vi "WS1050_AD7747_Control_Cap_bank_Measure S0.vi"(0 "Select Com Port":refnum<visa-resource-name>="COM1", 1 "Click down to quit":bool, 2 "Push Button to Initialize AD7747":bool, 3 "Push Button to Calibrate":bool, 7 "Push Button to write Offset":bool, 11 "errorin":errorcluster, 12 "Push Button to Measue Cap":bool=TRUE, 13 "CApDac_values":string[](array[string])=["900b89", "900b89", "900b89"]) -> (4 "C2L(pF)":dbl, 8 "C1L(pF)":dbl, 10 "C3L(pF)":dbl, 14 "Com Port Out":refnum<visa-resource-name>="COM1", 15 "error out":errorcluster)   [LabVIEW 2009]
panel:
  # "AD7747 Control Ver1.0"
  # "Interface PIC I2C Control"
  # "Bank Cap Measurements"
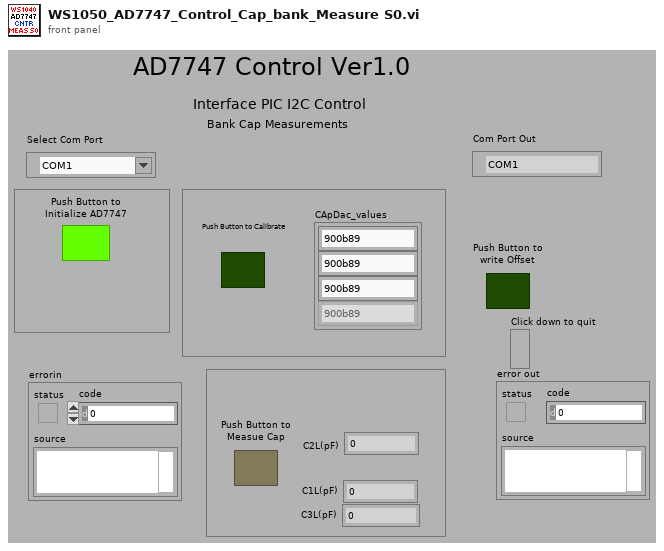
[diagram p1: front panel]
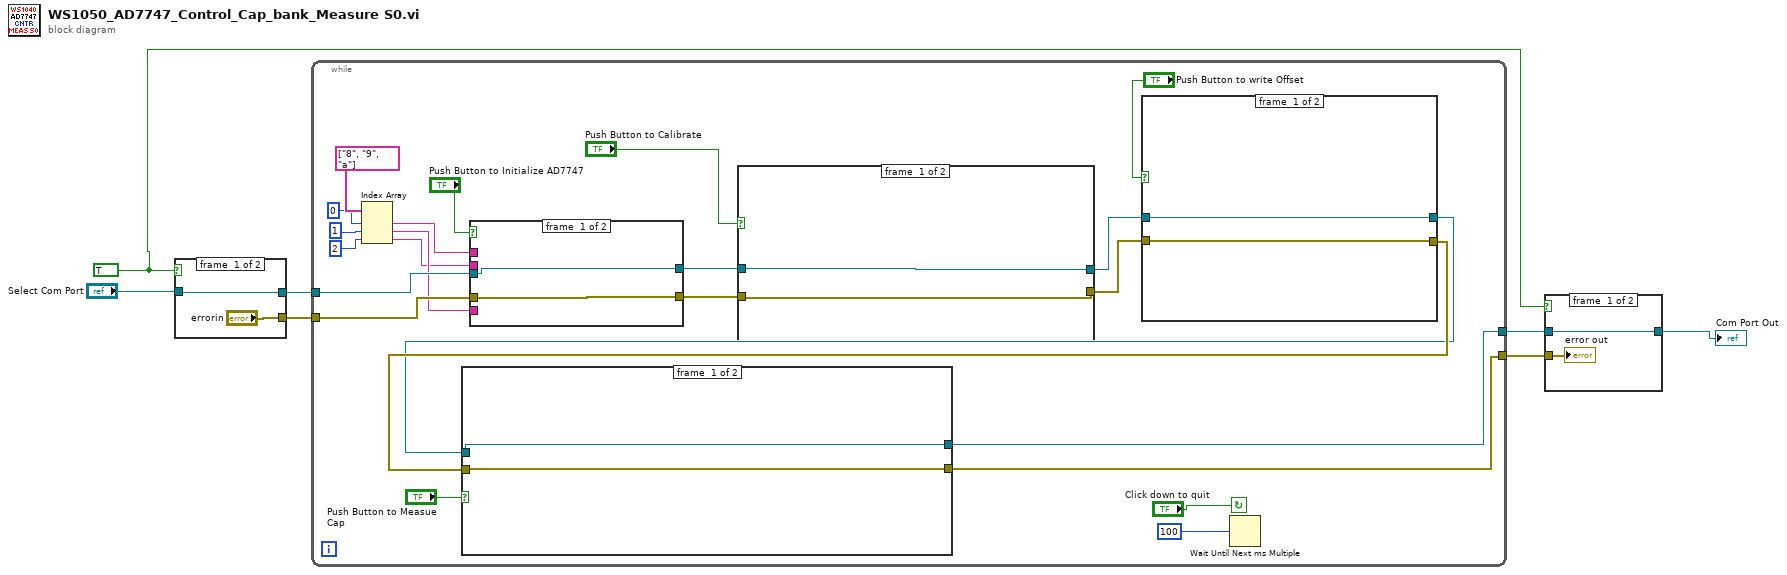
[diagram p0: block diagram]
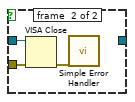
[diagram p2: hidden frame]
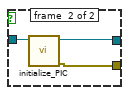
[diagram p3: hidden frame]
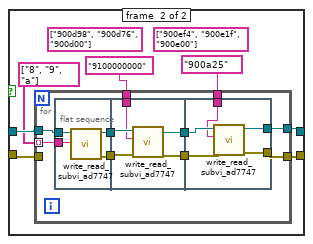
[diagram p4: hidden frame]
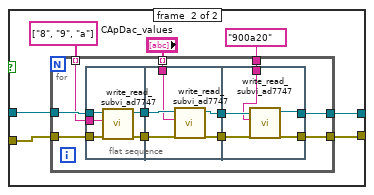
[diagram p5: hidden frame]
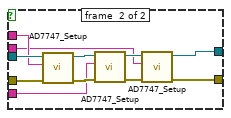
[diagram p6: hidden frame]
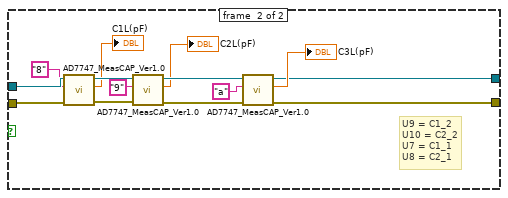
[diagram p7: hidden frame]
diagram:
  w2 = TRUE
  n1 = case shown="True" w2 {
    tunnel: ["errorin" w12] -> w7
    tunnel: [w8 w11] -> w6
    tunnel: "Select Com Port" -> [w8 w10]
    frame #0 {
    }
    frame #1 {
      n2 = call "initialize_PIC.vi"("Select Com Port"=w10) -> ("error out"=w12:errorcluster, "VISA resource name out"=w11:refnum<visa-resource-name>)  [unwired: 9 in]
    }
  }
  n3 = while {
    tunnel: w7 -> [w30]
    tunnel: w6 -> [w28]
    tunnel: [w17] -> w5
    tunnel: [w35] -> w4
    stop <- "Click down to quit" continue-if-true
    n4 = Index Array(array=string[] ["8", "9", "a"], index #1=0 ("index"), index #2=1 ("index"), index #3=2 ("index")) -> (element #1=w31:string, element #2=w24:string, element #3=w23:string)
    n5 = case shown="True" "Push Button to Initialize AD7747" {
      tunnel: w30 -> [w104 w115]
      tunnel: [w104 w105] -> w18
      tunnel: w28 -> [w103 w114]
      tunnel: w31 -> [_ w109]
      tunnel: w24 -> [_ w108]
      tunnel: w23 -> [_ w107]
      tunnel: [w103 w106] -> w15
      frame #0 {
      }
      frame #1 {
        n6 = call "AD7747_Setup.vi"("error in"=w115, "AD7747_Number"=w109, "Control"=w114) -> ("error out"=w113:errorcluster, "Control out"=w112:refnum<visa-resource-name>)  [unwired: 6 in, 1 out]
        n7 = call "AD7747_Setup.vi"("error in"=w113, "AD7747_Number"=w108, "Control"=w112) -> ("error out"=w111:errorcluster, "Control out"=w110:refnum<visa-resource-name>)  [unwired: 6 in, 1 out]
        n8 = call "AD7747_Setup.vi"("error in"=w111, "AD7747_Number"=w107, "Control"=w110) -> ("error out"=w105:errorcluster, "Control out"=w106:refnum<visa-resource-name>)  [unwired: 6 in, 1 out]
      }
    }
    n9 = case shown="True" "Push Button to Calibrate" {
      tunnel: [w69 w77] -> w29
      tunnel: w18 -> [w69 w74]
      tunnel: w15 -> [w70 w73]
      tunnel: [w70 w72] -> w14
      frame #0 {
      }
      frame #1 {
        n10 = for {
          tunnel: [w83] -> w77
          tunnel: w73 -> [w87]
          tunnel: w74 -> [w88]
          tunnel: string[] ["8", "9", "a"] -> [w86] mode=indexing
          tunnel: "CApDac_values" -> [w82] mode=indexing
          tunnel: [w81] -> w72
          tunnel: "900a20" ("Data_In 2") -> [w78]
          n11 = flat-sequence {
            tunnel: w88 -> [w93]
            tunnel: w87 -> [w91]
            tunnel: w86 -> [w89]
            tunnel: [w92] -> w85
            tunnel: [w90] -> w84
            tunnel: w85 -> [w97]
            tunnel: w84 -> [w98]
            tunnel: w82 -> [w95]
            tunnel: [w96] -> w80
            tunnel: [w94] -> w79
            tunnel: [w100] -> w81
            tunnel: [w102] -> w83
            tunnel: w80 -> [w102]
            tunnel: w79 -> [w101]
            tunnel: w78 -> [w99]
            frame #0 {
              n12 = call "write_read_subvi_ad7747.vi"("error in (no error)"=w93, "command"=w89, "Control"=w91) -> ("error out"=w92:errorcluster, "Control out"=w90:refnum<visa-resource-name>)  [unwired: 6 in, 1 out]
            }
            frame #1 {
              n13 = call "write_read_subvi_ad7747.vi"("error in (no error)"=w97, "command"=w95, "Control"=w98) -> ("error out"=w96:errorcluster, "Control out"=w94:refnum<visa-resource-name>)  [unwired: 6 in, 1 out]
            }
            frame #2 {
              n14 = call "write_read_subvi_ad7747.vi"("command"=w99, "Control"=w101) -> ("Control out"=w100:refnum<visa-resource-name>)  [unwired: 7 in, 2 out]
            }
          }
        }
      }
    }
    n15 = case shown="True" "Push Button to write Offset" {
      tunnel: w14 -> [w36 w43]
      tunnel: w29 -> [w37 w44]
      tunnel: [w37 w41] -> w16
      tunnel: [w36 w40] -> w13
      frame #0 {
      }
      frame #1 {
        (unwired) string[] ["900ef4", "900e1f", "900e00"]
        (unwired) string[] ["900d98", "900d76", "900d00"]
        n16 = for {
          tunnel: w44 -> [_]
          tunnel: [w48] -> w41
          tunnel: w43 -> [w54]
          tunnel: string[] ["8", "9", "a"] -> [w53] mode=indexing
          tunnel: "9100000000" ("Data_In 2") -> [w47]
          tunnel: "900a25" ("Data_In 2") -> [w46]
          tunnel: [w45] -> w40
          n17 = flat-sequence {
            tunnel: w54 -> [w56]
            tunnel: w53 -> [w55]
            tunnel: [w58] -> w52
            tunnel: [w57] -> w51
            tunnel: w52 -> [w61]
            tunnel: w51 -> [w63]
            tunnel: [w60] -> w50
            tunnel: [w62] -> w49
            tunnel: w47 -> [w59]
            tunnel: w50 -> [w67]
            tunnel: w49 -> [w68]
            tunnel: [w66] -> w48
            tunnel: w46 -> [w65]
            tunnel: [w64] -> w45
            frame #0 {
              n18 = call "write_read_subvi_ad7747.vi"("command"=w55, "Control"=w56) -> ("error out"=w58:errorcluster, "Control out"=w57:refnum<visa-resource-name>)  [unwired: 7 in, 1 out]
            }
            frame #1 {
              n19 = call "write_read_subvi_ad7747.vi"("error in (no error)"=w61, "command"=w59, "Control"=w63) -> ("error out"=w60:errorcluster, "Control out"=w62:refnum<visa-resource-name>)  [unwired: 6 in, 1 out]
            }
            frame #2 {
              n20 = call "write_read_subvi_ad7747.vi"("error in (no error)"=w67, "command"=w65, "Control"=w68) -> ("error out"=w66:errorcluster, "Control out"=w64:refnum<visa-resource-name>)  [unwired: 6 in, 1 out]
            }
          }
        }
      }
    }
    n21 = case shown="True" "Push Button to Measue Cap" {
      tunnel: w16 -> [w117 w131]
      tunnel: w13 -> [w116 w130]
      tunnel: [w117 w119] -> w17
      tunnel: [w116 w118] -> w35
      frame #0 {
      }
      frame #1 {
        # "U9 = C1_2\nU10 = C2_2\nU7 = C1_1\nU8 = C2_1"
        n22 = call "AD7747_MeasCAP_Ver1.0.vi"("error in (no error)"=w131, "AD7747_Number"="8", "Control"=w130) -> ("error"=w127:errorcluster, "CAP (pF)"=→"C1L(pF)":dbl, "Control out"=w126:refnum<visa-resource-name>)  [unwired: 5 in, 1 out]
        n23 = call "AD7747_MeasCAP_Ver1.0.vi"("error in (no error)"=w127, "AD7747_Number"="9", "Control"=w126) -> ("error"=w124:errorcluster, "CAP (pF)"=→"C2L(pF)":dbl, "Control out"=w123:refnum<visa-resource-name>)  [unwired: 5 in, 1 out]
        n24 = call "AD7747_MeasCAP_Ver1.0.vi"("error in (no error)"=w124, "AD7747_Number"="a", "Control"=w123) -> ("error"=w119:errorcluster, "CAP (pF)"=→"C3L(pF)":dbl, "Control out"=w118:refnum<visa-resource-name>)  [unwired: 5 in, 1 out]
      }
    }
    n25 = Wait Until Next ms Multiple(millisecond multiple=u32 100) -> ()  [unwired: 1 out]
  }
  n26 = case shown="True" w2 {
    tunnel: w5 -> [w133 w135]
    tunnel: w4 -> [w132 w134]
    tunnel: [w132 _] -> w1
    frame #0 {
      "error out" <- w133
    }
    frame #1 {
      n27 = VISA Close(VISA resource name=w134, error in (no error)=w135) -> (error out=w136:errorcluster)
      n28 = call <vilib>:"Simple Error Handler.vi"("error in (no error)"=w136) -> ()  [unwired: 1 in, 8 out]
    }
  }
  "Com Port Out" <- w1
